vi "Elmo Init SDO.vi"(8 "Error In":errorcluster caption="Error Out", 9 "Timeout(Scans)":i32=10000, 11 "Elmo Driver IO":refnum<k21>="ni.var.io://NI cRIO/EtherCAT Master/Device") -> (0 "error out":errorcluster)   [LabVIEW 2019]
uses:
  Elmo Init State.ctl
  <resource>/objmgr/IndComECAT.rc
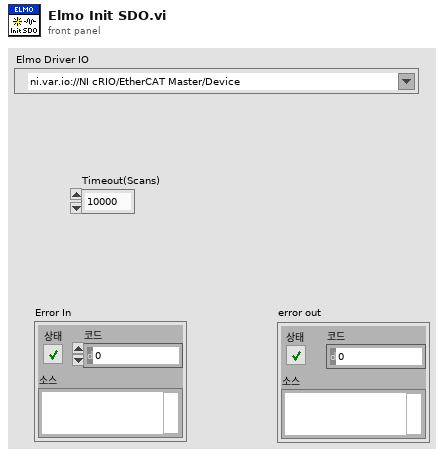
[diagram p1: front panel]
types:
  T1 = typedef "Elmo Init State.ctl" = enum16{"Check ECAT", "Set Init", "Set PreOP", "Set SafeOP", "Set OP", "Check Driver", "Set ready to switch on", "Set Operation Enabled", "Fault Reset", "Set Max Torque", "Set Current Mode", "Set Quick Stop Option", "Close"}
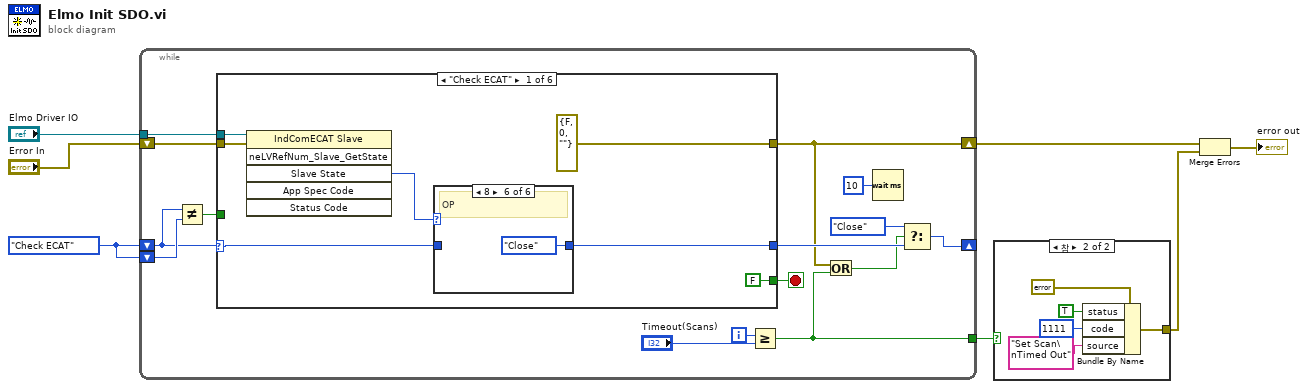
[diagram p0: block diagram]
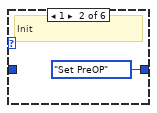
[diagram p3: hidden frame]
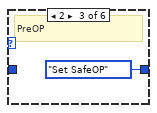
[diagram p4: hidden frame]
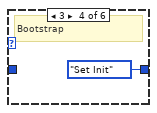
[diagram p5: hidden frame]
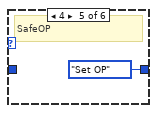
[diagram p6: hidden frame]
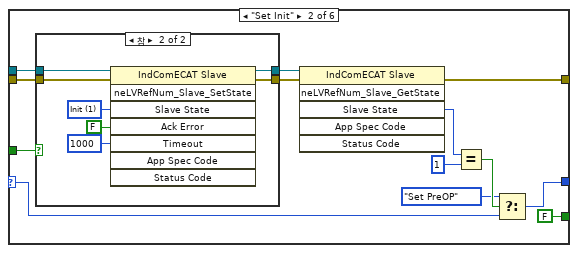
[diagram p7: hidden frame]
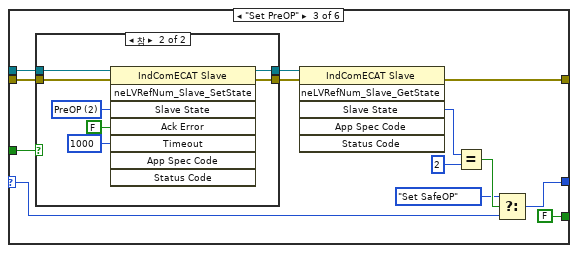
[diagram p9: hidden frame]
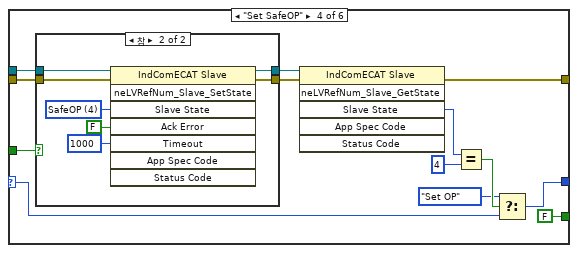
[diagram p11: hidden frame]
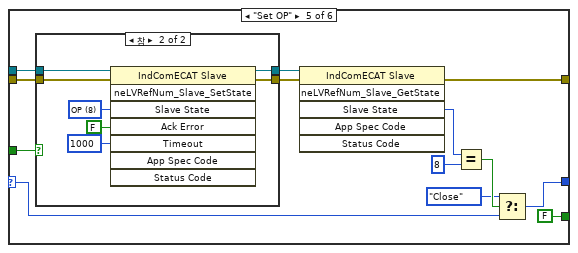
[diagram p13: hidden frame]
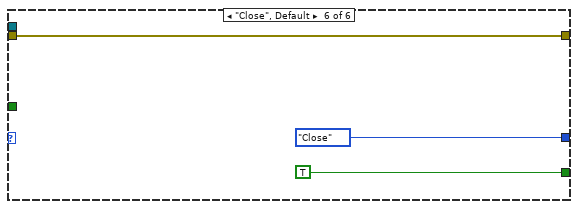
[diagram p15: hidden frame]
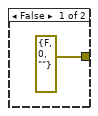
[diagram p16: hidden frame]
diagram:
  w7 = Elmo_Init_State."Check ECAT"
  n1 = while {
    shift-right: [w17] -> _
    shift-left: w7 -> [w8]
    shift-left: w7 -> [w22]
    shift-right: [w13] -> w2
    shift-left: "Error In" -> [w20]
    tunnel: [w11] -> w5
    tunnel: "Elmo Driver IO" -> [w10]
    i -> [w16]
    stop <- w14 stop-if-true
    n2 = Not Equal?(x=w8, y=w22) -> (x != y?=w21:bool)
    n3 = case shown="\"Check ECAT\"" w8 {
      selector: w8 -> [w25 w40 w62 w84 w106 _]
      tunnel: [w26 w38 w60 w82 w104 Elmo_Init_State."Close"] -> w19
      tunnel: w21 -> [_ w46 w68 w90 w112 _]
      tunnel: [errorcluster {"status"=FALSE, "code"=0, "source"=""} ("에러 출력") w37 w59 w81 w103 w126] -> w13
      tunnel: w20 -> [w27 w47 w69 w91 w113 w126]
      tunnel: [FALSE FALSE FALSE FALSE FALSE TRUE] -> w14
      tunnel: w10 -> [w29 w48 w70 w92 w114 _]
      frame "Check ECAT" {
        n4 = invoke class="IndComECAT Slave" method="neLVRefNum_Slave_GetState"(reference=w29, error in=w27) -> ("Slave State"=w28:u32)  [unwired: 4 in, 5 out]
        n5 = case shown="8" w28 {
          tunnel: [w30 Elmo_Init_State."Set PreOP" Elmo_Init_State."Set SafeOP" Elmo_Init_State."Set Init" Elmo_Init_State."Set OP" Elmo_Init_State."Close"] -> w26
          tunnel: w25 -> [w30 _ _ _ _ _]
          frame 0, Default {
            # "Unknown"
          }
          frame 1 {
            # "Init"
          }
          frame 2 {
            # "PreOP"
          }
          frame 3 {
            # "Bootstrap"
          }
          frame 4 {
            # "SafeOP"
          }
          frame 8 {
            # "OP"
          }
        }
      }
      frame "Set Init" {
        n6 = case shown="참" w46 {
          tunnel: w48 -> [w50 w56]
          tunnel: w47 -> [w49 w55]
          tunnel: [w50 w54] -> w45
          tunnel: [w49 w53] -> w44
          frame False {
          }
          frame True {
            w57 = u32 1 items=["Init"=1, "PreOP"=2, "BootStrap"=3, "SafeOP"=4, "OP"=8] ("Slave State")
            n7 = invoke class="IndComECAT Slave" method="neLVRefNum_Slave_SetState"(reference=w56, error in=w55, "Slave State"=w57, "Ack Error"=FALSE, "Timeout"=u32 1000) -> (reference out=w54:refnum<k21>, error out=w53:errorcluster)  [unwired: 3 in, 6 out]
          }
        }
        n8 = invoke class="IndComECAT Slave" method="neLVRefNum_Slave_GetState"(reference=w45, error in=w44) -> (error out=w37:errorcluster, "Slave State"=w43:u32)  [unwired: 4 in, 4 out]
        n9 = Equal?(x=w43, y=u32 1) -> (x = y?=w41:bool)
        n10 = Select(t=Elmo_Init_State."Set PreOP", s=w41, f=w40) -> (s? t:f=w38:T1)
      }
      frame "Set PreOP" {
        n11 = case shown="참" w68 {
          tunnel: w70 -> [w72 w78]
          tunnel: w69 -> [w71 w77]
          tunnel: [w72 w76] -> w67
          tunnel: [w71 w75] -> w66
          frame False {
          }
          frame True {
            w79 = u32 2 items=["Init"=1, "PreOP"=2, "BootStrap"=3, "SafeOP"=4, "OP"=8] ("Slave State")
            n12 = invoke class="IndComECAT Slave" method="neLVRefNum_Slave_SetState"(reference=w78, error in=w77, "Slave State"=w79, "Ack Error"=FALSE, "Timeout"=u32 1000) -> (reference out=w76:refnum<k21>, error out=w75:errorcluster)  [unwired: 3 in, 6 out]
          }
        }
        n13 = invoke class="IndComECAT Slave" method="neLVRefNum_Slave_GetState"(reference=w67, error in=w66) -> (error out=w59:errorcluster, "Slave State"=w65:u32)  [unwired: 4 in, 4 out]
        n14 = Equal?(x=w65, y=u32 2) -> (x = y?=w63:bool)
        n15 = Select(t=Elmo_Init_State."Set SafeOP", s=w63, f=w62) -> (s? t:f=w60:T1)
      }
      frame "Set SafeOP" {
        n16 = case shown="참" w90 {
          tunnel: w92 -> [w94 w100]
          tunnel: w91 -> [w93 w99]
          tunnel: [w94 w98] -> w89
          tunnel: [w93 w97] -> w88
          frame False {
          }
          frame True {
            w101 = u32 4 items=["Init"=1, "PreOP"=2, "BootStrap"=3, "SafeOP"=4, "OP"=8] ("Slave State")
            n17 = invoke class="IndComECAT Slave" method="neLVRefNum_Slave_SetState"(reference=w100, error in=w99, "Slave State"=w101, "Ack Error"=FALSE, "Timeout"=u32 1000) -> (reference out=w98:refnum<k21>, error out=w97:errorcluster)  [unwired: 3 in, 6 out]
          }
        }
        n18 = invoke class="IndComECAT Slave" method="neLVRefNum_Slave_GetState"(reference=w89, error in=w88) -> (error out=w81:errorcluster, "Slave State"=w87:u32)  [unwired: 4 in, 4 out]
        n19 = Equal?(x=w87, y=u32 4) -> (x = y?=w85:bool)
        n20 = Select(t=Elmo_Init_State."Set OP", s=w85, f=w84) -> (s? t:f=w82:T1)
      }
      frame "Set OP" {
        n21 = case shown="참" w112 {
          tunnel: w114 -> [w116 w122]
          tunnel: w113 -> [w115 w121]
          tunnel: [w116 w120] -> w111
          tunnel: [w115 w119] -> w110
          frame False {
          }
          frame True {
            w123 = u32 8 items=["Init"=1, "PreOP"=2, "BootStrap"=3, "SafeOP"=4, "OP"=8] ("Slave State")
            n22 = invoke class="IndComECAT Slave" method="neLVRefNum_Slave_SetState"(reference=w122, error in=w121, "Slave State"=w123, "Ack Error"=FALSE, "Timeout"=u32 1000) -> (reference out=w120:refnum<k21>, error out=w119:errorcluster)  [unwired: 3 in, 6 out]
          }
        }
        n23 = invoke class="IndComECAT Slave" method="neLVRefNum_Slave_GetState"(reference=w111, error in=w110) -> (error out=w103:errorcluster, "Slave State"=w109:u32)  [unwired: 4 in, 4 out]
        n24 = Equal?(x=w109, y=u32 8) -> (x = y?=w107:bool)
        n25 = Select(t=Elmo_Init_State."Close", s=w107, f=w106) -> (s? t:f=w104:T1)
      }
      frame "Close", Default {
      }
    }
    n26 = Greater Or Equal?(x=w16, y="Timeout(Scans)") -> (x >= y?=w11:bool)
    n27 = Or(x=w13, y=w11) -> (x .or. y?=w12:bool)
    n28 = Wait (ms)(milliseconds to wait=u32 10 ("대기 시간(ms)")) -> ()  [unwired: 1 out]
    n29 = Select(t=Elmo_Init_State."Close", s=w12, f=w19) -> (s? t:f=w17:T1)
  }
  n30 = case shown="참" w5 {
    tunnel: [errorcluster {"status"=FALSE, "code"=0, "source"=""} ("error out") w128] -> w6
    frame False {
    }
    frame True {
      n31 = Bundle By Name(cluster=errorcluster {"status"=FALSE, "code"=0, "source"=""} ("error out"), "status"=TRUE, "code"=1111, "source"="Set Scan\nTimed Out") -> (w128:errorcluster)
    }
  }
  n32 = Merge Errors(w2, w6) -> (→"error out":errorcluster)
